vi "Inst_DS360.vi"(8 "error in":errorcluster, 10 "All Message Queues in":T1, 11 "Prueba04 in":refnum<class "Prueba04.lvclass">) -> (0 "error out":errorcluster)   [LabVIEW 2019, in "Prueba04.lvclass"]
uses:
  Prueba04.lvclass
  QMH/Message Queue/All Message Queues.ctl
  QMH/Message Queue/Message Cluster.ctl
  Prueba04.lvclass/Prueba04.ctl
  Control/SetPointGEN.ctl
  <vilib>/Utility/error.llb/Error Cluster From Error Code.vi
  QMH/Message Queue/Enqueue Message (Single).vi
  <vilib>/ErrorRing/Error Ring.xnode
  QMH/Message Queue/Message Queue.lvlib
  Instrumento/DS360/DS360.lvclass
panel:
  out "All States":string[](array[string])
  out "Actual State":string
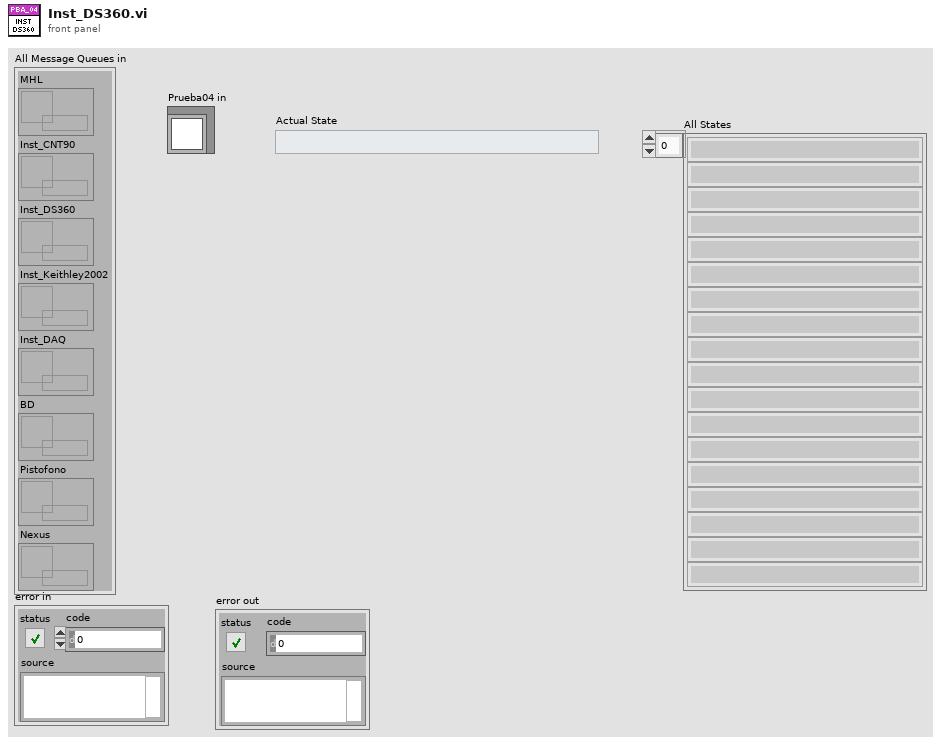
[diagram p1: front panel]
types:
  T1 = typedef "Message Queue.lvlib/All Message Queues.ctl" = cluster{"MHL":refnum<queue>, "Inst_CNT90":refnum<queue>, "Inst_DS360":refnum<queue>, "Inst_Keithley2002":refnum<queue>, "Inst_DAQ":refnum<queue>, "BD":refnum<queue>, "Pistofono":refnum<queue>, "Nexus":refnum<queue>}
  T2 = typedef "Prueba04.lvclass/SetPointGEN.ctl" = cluster{"frec":dbl, "amp":dbl, "letra":string}
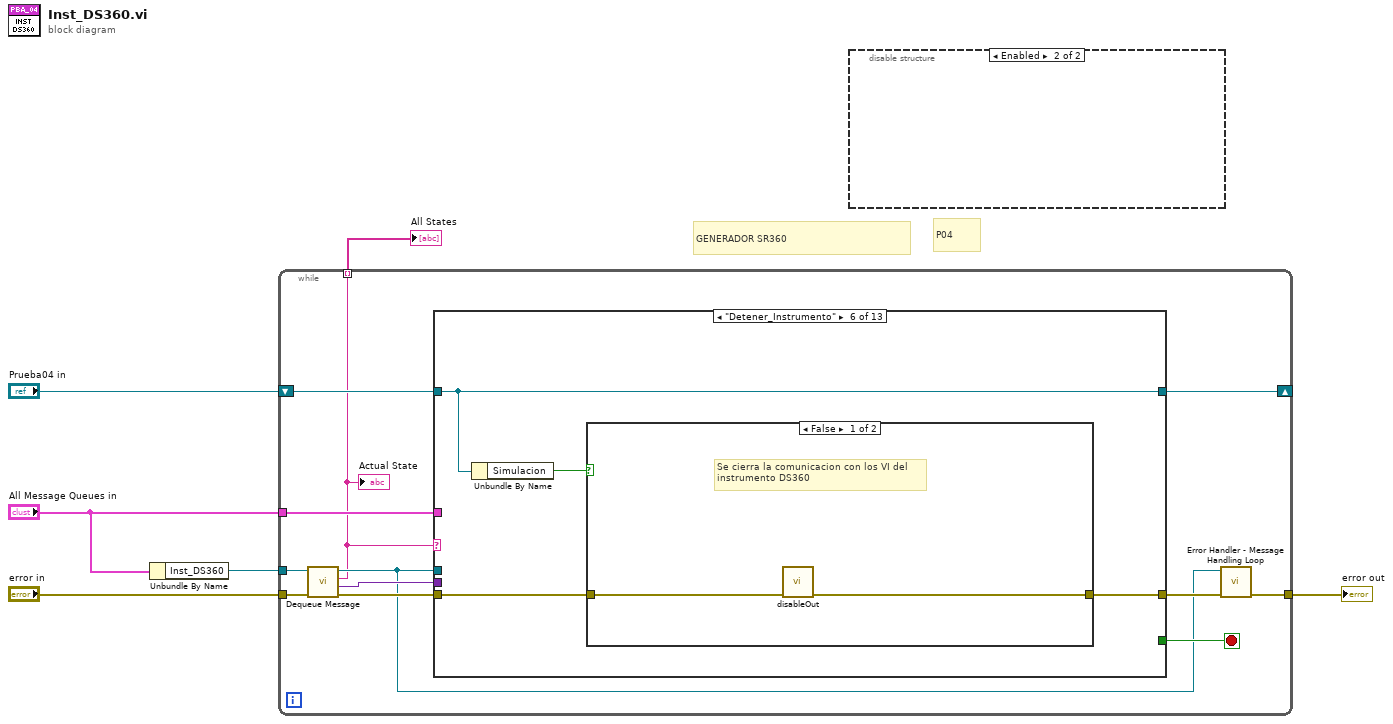
[diagram p0: block diagram]
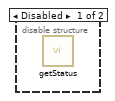
[diagram p2: hidden frame]
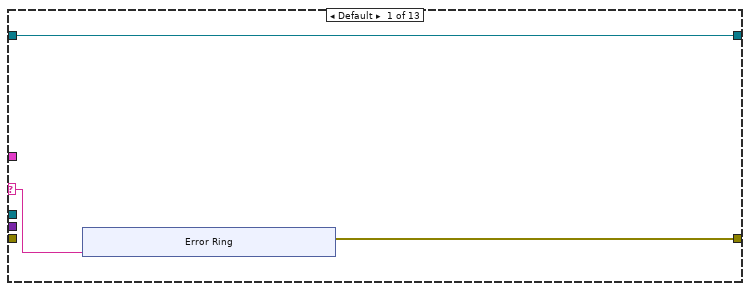
[diagram p3: hidden frame]
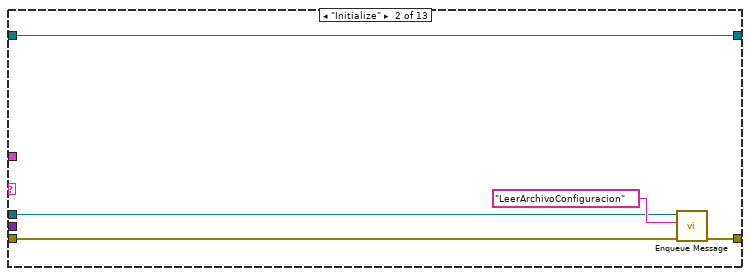
[diagram p4: hidden frame]
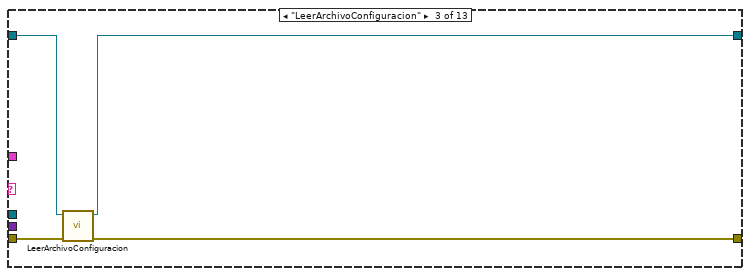
[diagram p5: hidden frame]
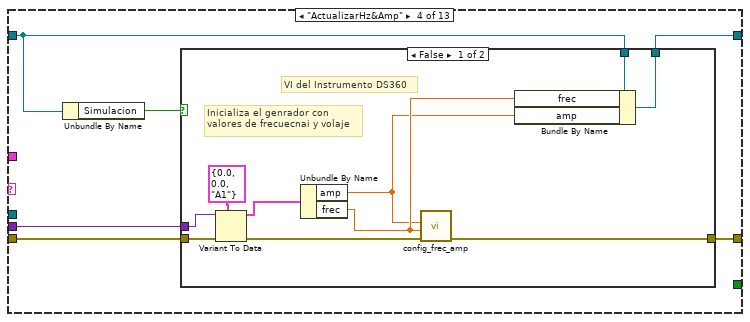
[diagram p6: hidden frame]
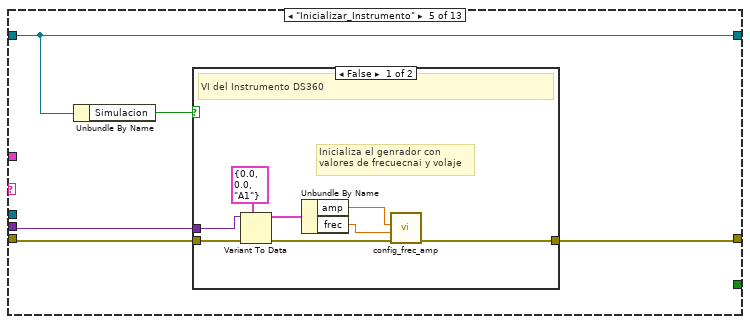
[diagram p8: hidden frame]
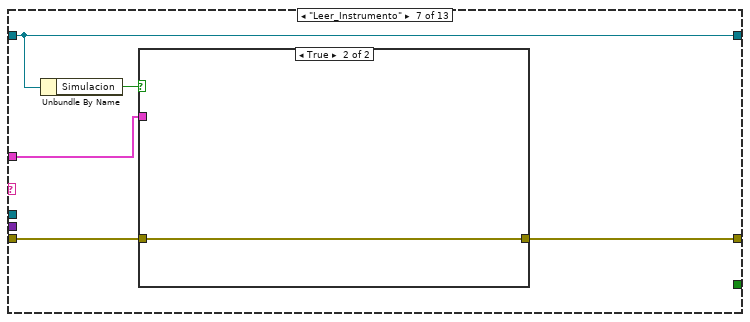
[diagram p11: hidden frame]
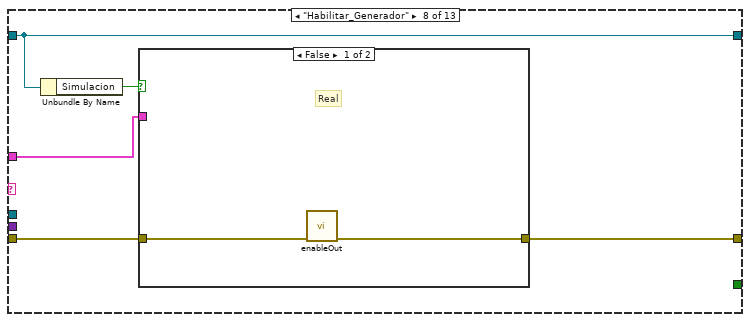
[diagram p13: hidden frame]
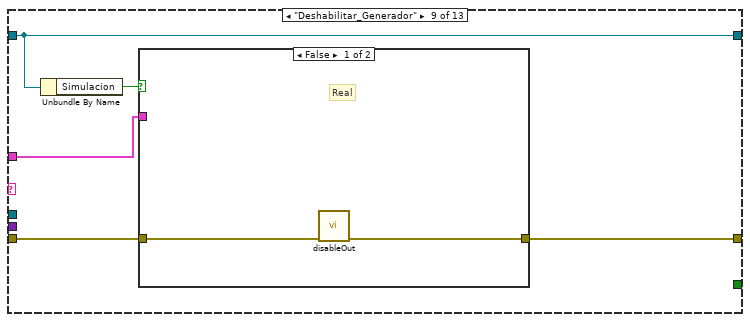
[diagram p15: hidden frame]
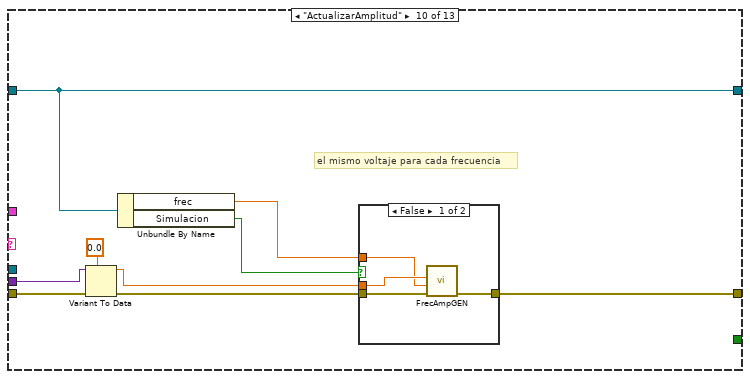
[diagram p17: hidden frame]
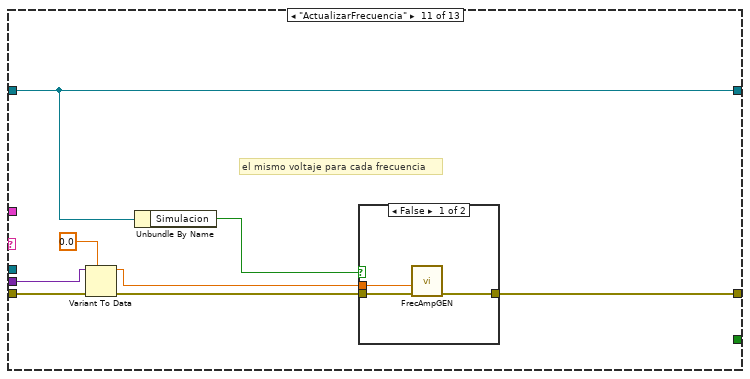
[diagram p19: hidden frame]
diagram:
  # "P04"
  # "GENERADOR SR360"
  n1 = Unbundle By Name("All Message Queues in") -> ("Inst_DS360"=w4:refnum<queue>)
  n2 = while {
    tunnel: "error in" -> [w18]
    tunnel: w4 -> [w17]
    tunnel: "All Message Queues in" -> [w16]
    tunnel: [w9] -> w2
    shift-right: [w12] -> _
    shift-left: "Prueba04 in" -> [w15]
    tunnel: [w7] -> w1 mode=indexing
    stop <- w11 stop-if-true
    n3 = call "Dequeue Message.vi"("error in (no error)"=w18, "Message Queue"=w17) -> ("error out"=w13:errorcluster, "Message Data"=w14:variant, "Message"=w7:string, "dup Message Queue"=w8:refnum<queue>)  [unwired: 6 in]
    "Actual State" <- w7
    n4 = case shown="\"Detener_Instrumento\"" w7 {
      selector: w7 -> [w21 _ _ _ _ _ _ _ _ _ _ w128 _]
      tunnel: w16 -> [_ _ _ _ _ _ w80 w87 w95 _ _ w127 _]
      tunnel: w15 -> [w19 w33 w34 w39 w57 w72 w79 w86 w94 w104 w117 w135 w137]
      tunnel: w8 -> [_ w29 _ _ _ _ _ _ _ _ _ _ w139]
      tunnel: w14 -> [_ _ _ w41 w58 _ _ _ _ w105 w118 w132 _]
      tunnel: w13 -> [_ w30 w36 w40 w59 w70 w81 w88 w96 w106 w119 w133 w140]
      tunnel: [w20 w31 w37 w43 w56 w73 w77 w84 w92 w108 w121 w130 w136] -> w10
      tunnel: [w19 w33 w35 w38 w57 w72 w79 w86 w94 w104 w117 w135 w137] -> w12
      tunnel: [_ _ _ _ _ _ _ _ _ _ _ _ TRUE] -> w11
      frame Default {
        n5 = xnode "Error Ring"("parameter 0"=w21) -> ("error out"=w20:errorcluster)
      }
      frame "Initialize" {
        n6 = call-poly "Enqueue Message.vi"("error in (no error)"=w30, "Message"="LeerArchivoConfiguracion", "Message Queue"=w29) -> ("error out"=w31:errorcluster)  [unwired: 7 in, 1 out]
      }
      frame "LeerArchivoConfiguracion" {
        n7 = call "LeerArchivoConfiguracion.vi"("error in (no error)"=w36, "Prueba04 in"=w34) -> ("error out"=w37:errorcluster, "Prueba04 out"=w35:refnum<class "Prueba04.lvclass">)  [unwired: 8 in]
      }
      frame "ActualizarHz&Amp" {
        n8 = Unbundle By Name(w39) -> ("Simulacion"=w42:bool)
        n9 = case shown="False" w42 {
          tunnel: [w52 w55] -> w43
          tunnel: w40 -> [w53 w55]
          tunnel: w41 -> [w50 _]
          tunnel: w39 -> [w47 w54]
          tunnel: [w44 w54] -> w38
          frame False {
            # "Inicializa el genrador con \nvalores de frecuecnai y volaje"
            # "VI del Instrumento DS360"
            n10 = Variant To Data(error in=w53, type=T2 {"frec"=0.0, "amp"=0.0, "letra"="A1"} ("setpoint"), Variant=w50) -> (data=w48:T2, error out=w51:errorcluster)
            n11 = Unbundle By Name(w48) -> ("amp"=w45:dbl, "frec"=w46:dbl)
            n12 = call "config_frec_amp.vi"("error in (no error)"=w51, "Frec (Hz)"=w46, "Amplitud (Vrms)"=w45) -> ("error out"=w52:errorcluster)  [unwired: 7 in, 1 out]
            n13 = Bundle By Name(cluster=w47, "frec"=w46, "amp"=w45) -> (w44:refnum<class "Prueba04.lvclass">)
          }
          frame True {
            # "Simulacion"
          }
        }
      }
      frame "Inicializar_Instrumento" {
        n14 = Unbundle By Name(w57) -> ("Simulacion"=w60:bool)
        n15 = case shown="False" w60 {
          tunnel: [w67 w69] -> w56
          tunnel: w59 -> [w68 w69]
          tunnel: w58 -> [w65 _]
          frame False {
            # "Inicializa el genrador con \nvalores de frecuecnai y volaje"
            # "VI del Instrumento DS360"
            n16 = Variant To Data(error in=w68, type=T2 {"frec"=0.0, "amp"=0.0, "letra"="A1"}, Variant=w65) -> (data=w63:T2, error out=w66:errorcluster)
            n17 = Unbundle By Name(w63) -> ("amp"=w62:dbl, "frec"=w61:dbl)
            n18 = call "config_frec_amp.vi"("error in (no error)"=w66, "Frec (Hz)"=w61, "Amplitud (Vrms)"=w62) -> ("error out"=w67:errorcluster)  [unwired: 7 in, 1 out]
          }
          frame True {
            # "Simulacion"
          }
        }
      }
      frame "Detener_Instrumento" {
        n19 = Unbundle By Name(w72) -> ("Simulacion"=w71:bool)
        n20 = case shown="False" w71 {
          tunnel: [w75 w76] -> w73
          tunnel: w70 -> [w74 w76]
          frame False {
            # "Se cierra la comunicacion con los VI del\ninstrumento DS360"
            n21 = call "disableOut.vi"("error in (no error)"=w74) -> ("error out"=w75:errorcluster)  [unwired: 9 in, 1 out]
          }
          frame True {
            # "Simulacion"
          }
        }
      }
      frame "Leer_Instrumento" {
        n22 = Unbundle By Name(w79) -> ("Simulacion"=w78:bool)
        n23 = case shown="True" w78 {
          tunnel: [w82 w83] -> w77
          tunnel: w81 -> [w82 w83]
          tunnel: w80 -> [_ _]
          frame False {
          }
          frame True {
          }
        }
      }
      frame "Habilitar_Generador" {
        n24 = Unbundle By Name(w86) -> ("Simulacion"=w85:bool)
        n25 = case shown="False" w85 {
          tunnel: [w89 w91] -> w84
          tunnel: w88 -> [w90 w91]
          tunnel: w87 -> [_ _]
          frame False {
            # "Real"
            n26 = call "enableOut.vi"("error in (no error)"=w90) -> ("error out"=w89:errorcluster)  [unwired: 9 in, 1 out]
          }
          frame True {
            # "Simulacion"
          }
        }
      }
      frame "Deshabilitar_Generador" {
        n27 = Unbundle By Name(w94) -> ("Simulacion"=w93:bool)
        n28 = case shown="False" w93 {
          tunnel: [w97 w99] -> w92
          tunnel: w96 -> [w98 w99]
          tunnel: w95 -> [_ _]
          frame False {
            # "Real"
            n29 = call "disableOut.vi"("error in (no error)"=w98) -> ("error out"=w97:errorcluster)  [unwired: 9 in, 1 out]
          }
          frame True {
            # "Simulacion"
          }
        }
      }
      frame "ActualizarAmplitud" {
        # "el mismo voltaje para cada frecuencia"
        n30 = Variant To Data(error in=w106, type=0.0, Variant=w105) -> (data=w102:dbl, error out=w107:errorcluster)
        n31 = Unbundle By Name(w104) -> ("frec"=w100:dbl, "Simulacion"=w101:bool)
        n32 = case shown="False" w101 {
          tunnel: [w112 w113] -> w108
          tunnel: w107 -> [w111 w113]
          tunnel: w102 -> [w110 _]
          tunnel: w100 -> [w109 _]
          frame False {
            n33 = call "FrecAmpGEN.vi"("error in (no error)"=w111, "Frec (Hz)"=w109, "Amplitud (Vrms)"=w110) -> ("error out"=w112:errorcluster)  [unwired: 7 in, 1 out]
          }
          frame True {
            # "Simlacion"
          }
        }
      }
      frame "ActualizarFrecuencia" {
        # "el mismo voltaje para cada frecuencia"
        n34 = Variant To Data(error in=w119, type=0.0, Variant=w118) -> (data=w115:dbl, error out=w120:errorcluster)
        n35 = Unbundle By Name(w117) -> ("Simulacion"=w114:bool)
        n36 = case shown="False" w114 {
          tunnel: [w124 w125] -> w121
          tunnel: w120 -> [w123 w125]
          tunnel: w115 -> [w122 _]
          frame False {
            n37 = call "FrecAmpGEN.vi"("error in (no error)"=w123, "Frec (Hz)"=w122) -> ("error out"=w124:errorcluster)  [unwired: 8 in, 1 out]
          }
          frame True {
            # "Simlacion"
          }
        }
      }
      frame "Error" {
        n38 = Unbundle By Name(w127) -> ("MHL"=w126:refnum<queue>)
        n39 = Variant To Data(error in=w133, type=errorcluster {"status"=FALSE, "code"=0, "source"=""} ("error constant"), Variant=w132) -> (data=w129:errorcluster, error out=w131:errorcluster)
        n40 = call-poly "Enqueue Message.vi"("error in (no error)"=w131, "Message Data"=w129, "Message"=w128, "Message Queue"=w126) -> ("error out"=w130:errorcluster)  [unwired: 6 in, 1 out]
      }
      frame "Exit" {
        n41 = Release Queue(queue=w139, error in (no error)=w140) -> (error out=w136:errorcluster)  [unwired: 1 in, 2 out]
      }
    }
    n42 = call "Error Handler - Message Handling Loop.vi"("error in (no error)"=w10, "Message Queue"=w8) -> ("dup error in"=w9:errorcluster)  [unwired: 8 in, 1 out]
  }
  "error out" <- w2
  "All States" <- w1
  n43 = disable-structure shown="Enabled" {
    frame Disabled {
      n44 = call "getStatus.vi"() -> ()  [unwired: 9 in, 3 out]
    }
    frame Enabled {
    }
  }
